vi "PatchSystemDefinitionFile.vi"(8 "error in (no error)":errorcluster, 11 "VeriStand Test Case in":refnum<class "VeriStandTestCase.lvclass">) -> (0 "error out":errorcluster, 3 "VeriStand Test Case out":refnum<class "VeriStandTestCase.lvclass">)   [LabVIEW 2027, in "VeriStandTestCase.lvclass"]
uses:
  VeriStandTestCase.lvclass
  VeriStandTestCase.lvclass/VeriStandTestCase.ctl
  VeriStandTestUtilities/VeriStandTestUtilities.lvlib
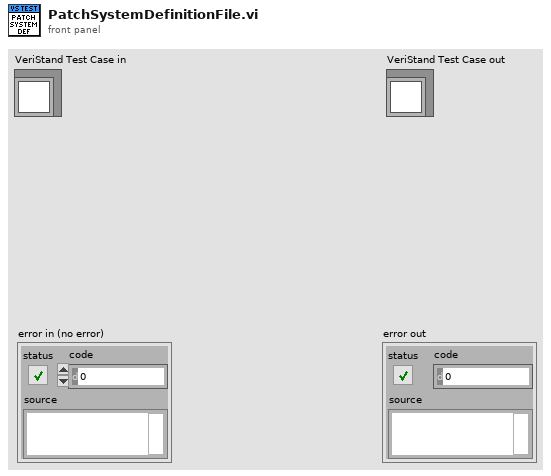
[diagram p1: front panel]
types:
  T1 = typedef "VeriStandTestUtilities.lvlib/ConfigOverrideItem.ctl" = cluster{"node":string, "property":string, "value":string}
  T2 = typedef "VeriStandTestUtilities.lvlib/TargetsConfiguration.ctl" = cluster{"Supported Targets":cluster{"IP Address / Hostname":string, "Target Platform":T3}[], "Active Configuration":T3}
  T3 = typedef "VeriStandTestUtilities.lvlib/TargetPlatform.ctl" = enum16{"Windows", "Linux64CRIO", "Linux64PXI", "LinuxARM", "PharLap"}
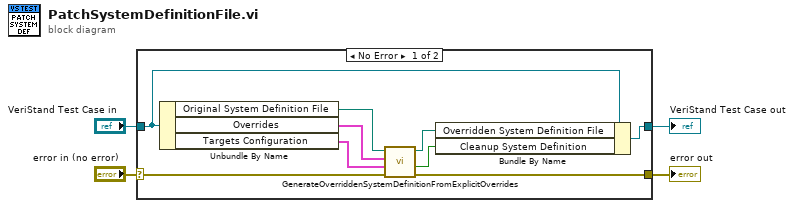
[diagram p0: block diagram]
diagram:
  n1 = case shown="No Error" "error in (no error)" {
    selector: "error in (no error)" -> [w9 w15]
    tunnel: [w13 w15] -> w4
    tunnel: "VeriStand Test Case in" -> [w10 w14]
    tunnel: [w12 w14] -> w1
    frame No Error {
      n2 = Unbundle By Name(w10) -> ("Original System Definition File"=w8:path, "Overrides"=w6:T1[], "Targets Configuration"=w5:T2)
      n3 = call "GenerateOverriddenSystemDefinitionFromExplicitOverrides.vi"("error in (no error)"=w9, "Targets Configuration"=w5, "overrides"=w6, "absolute system definition file"=w8) -> ("error out"=w13:errorcluster, "Temporary File?"=w11:bool, "absolute overridden system definition file"=w7:path)  [unwired: 5 in]
      n4 = Bundle By Name(cluster=w10, "Overridden System Definition File"=w7, "Cleanup System Definition"=w11) -> (w12:refnum<class "VeriStandTestCase.lvclass">)
    }
    frame Error {
    }
  }
  "error out" <- w4
  "VeriStand Test Case out" <- w1
